vi "GetAvgFulfillmentTime.vi"(8 "error in":errorcluster, 9 "To":timestamp, 10 "From":timestamp, 11 "PersonnelType":string="Dr") -> (0 "error out":errorcluster, 2 "AvgFulfillTime(s)":dbl)   [LabVIEW 2015, in "DatabaseApi.lvlib"]
uses:
  TypeDef/Request/RequestsFilter.ctl
  TypeDef/Request/RequestsTableColumnNamesRing.ctl
  DatabaseApi.lvlib
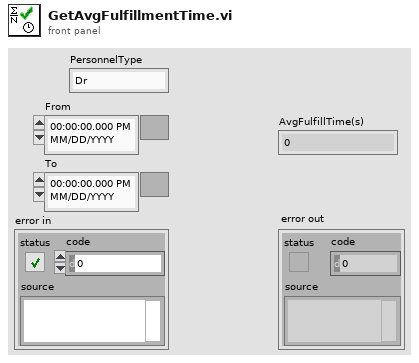
[diagram p1: front panel]
types:
  T1 = typedef "DatabaseApi.lvlib/RequestsTableColumnNamesRing.ctl" = enum16{"RequestID", "PersonnelType", "StartTime", "StartName", "AckTime", "AckName", "FulfilledTime", "FulfilledName", "Description", "Room Number", "Request Type", "Alarm"}
  T2 = typedef "DatabaseApi.lvlib/RequestsFilter.ctl" = cluster{"Filter":T1, "From":timestamp, "To":timestamp, "Filter Text":string, "Enable Filter":bool}
  T3 = typedef "Request.lvclass/RequestCluster.ctl" = cluster{"RequestID":string, "PersonelType":T4, "StartTime":timestamp, "StartName":string, "AckTime":timestamp, "AckName":string, "FulfilledTime":timestamp, "FulfilledName":string, "Description":string, "Room Number":i32, "Request Type":T5, "Alarm":bool}
  T4 = typedef "Request.lvclass/PersonnelType.ctl" = u16
  T5 = typedef "Request.lvclass/RequestType.ctl" = enum16{"Specific Call To Room", "General Call To Room"}
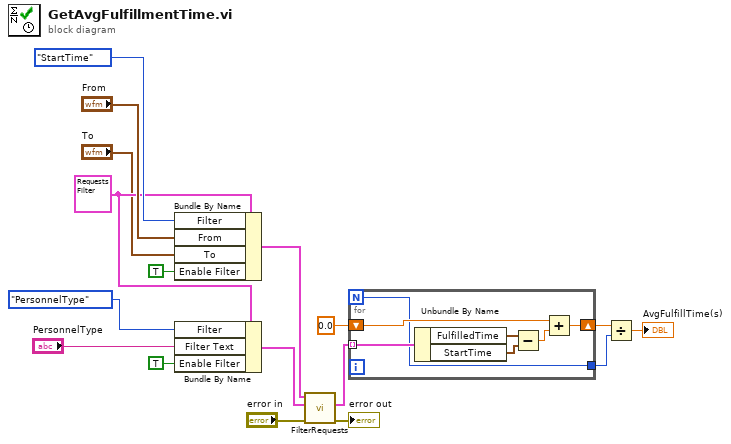
[diagram p0: block diagram]
diagram:
  w12 = T2 {"Filter"=enum."StartTime", "From"=timestamp(0 s since 1904-01-01), "To"=timestamp(0 s since 1904-01-01), "Filter Text"="", "Enable Filter"=FALSE} ("Filter 3")
  n1 = Bundle By Name(cluster=w12, "Filter"=RequestsTableColumnNamesRing."StartTime", "From"="From", "To"="To", "Enable Filter"=TRUE) -> (w15:T2)
  n2 = Bundle By Name(cluster=w12, "Filter"=RequestsTableColumnNamesRing."PersonnelType", "Filter Text"="PersonnelType", "Enable Filter"=TRUE) -> (w10:T2)
  n3 = call "FilterRequests.vi"("error in"="error in", "Filter 2"=w10, "Filter 1"=w15) -> ("error out"=→"error out":errorcluster, "Requests"=w7:T3[])  [unwired: 7 in]
  n4 = for {
    N -> [w19]
    tunnel: w7 -> [w24] mode=indexing
    shift-right: [w18] -> w5
    shift-left: 0.0 -> [w20]
    tunnel: [w19] -> w4
    n5 = Unbundle By Name(w24) -> ("FulfilledTime"=w23:timestamp, "StartTime"=w22:timestamp)
    n6 = Subtract(x=w23, y=w22) -> (x-y=w21:dbl)
    n7 = Add(x=w20, y=w21) -> (x+y=w18:dbl)
  }
  n8 = Divide(x=w5, y=w4) -> (x/y=→"AvgFulfillTime(s)":dbl)
